vi "Launch p2.vi"(9 "Alias":string, 10 "Actor":refnum<class "Actor.lvclass">, 11 "jettl in":refnum<class "jettl.lvclass">) -> (0 "error out":errorcluster)   [LabVIEW 2021, in "jettl.lvlib" / "jettl.lvclass"]
uses:
  jettl.lvclass
  Actor/Actor/Actor.lvclass
  Create Wrapper.vi
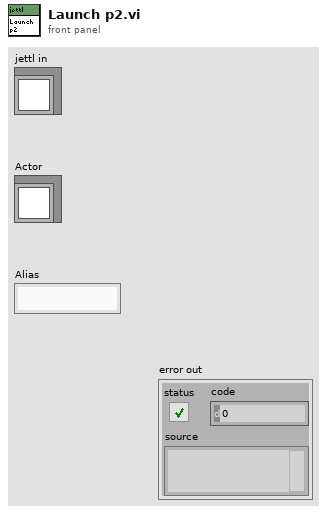
[diagram p1: front panel]
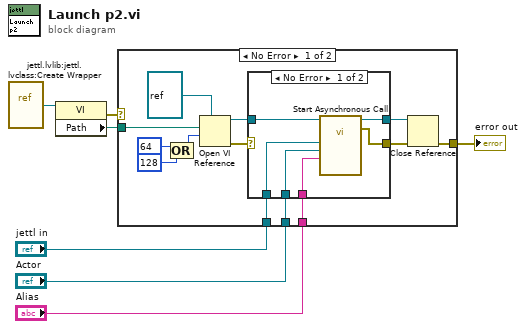
[diagram p0: block diagram]
diagram:
  n1 = vi-ref "jettl.lvlib:jettl.lvclass:Create Wrapper.vi"() -> (w6:refnum<vi>)
  n2 = property class="VI"(reference=w6) -> (error out=w7:errorcluster, "Path"=w5:path)  [unwired: 1 in, 1 out]
  n3 = case shown="No Error" w7 {
    selector: w7 -> [_ w29]
    tunnel: [w18 w29] -> w2
    tunnel: w5 -> [w14 _]
    tunnel: "Alias" -> [w10 _]
    tunnel: "Actor" -> [w9 _]
    tunnel: "jettl in" -> [w8 _]
    frame No Error {
      n4 = Compound Arithmetic op=OR(64 ("options: Multiple Clones,\n  Fire & Forget"), 128 ("options: Multiple Clones,\n  Fire & Forget")) -> (w16:i32)
      n5 = Open VI Reference(type specifier VI Refnum (for type only)=refnum<vi> refnum, vi path=w14, options=w16) -> (vi reference=w12:refnum<vi>, error out=w13:errorcluster)  [unwired: 3 in]
      n6 = case shown="No Error" w13 {
        selector: w13 -> [_ w28]
        tunnel: [w26 w27] -> w20
        tunnel: [w25 w28] -> w19
        tunnel: w12 -> [w24 w27]
        tunnel: w10 -> [w23 _]
        tunnel: w9 -> [w22 _]
        tunnel: w8 -> [w21 _]
        frame No Error {
          n7 = call-by-ref "Start Asynchronous Call"(reference=w24, "Alias"=w23, "Actor"=w22, "jettl in"=w21) -> (reference out=w26:refnum<vi>, error out=w25:errorcluster)  [unwired: 9 in, 1 out]
        }
        frame Error {
        }
      }
      n8 = Close Reference(reference=w20, error in (no error)=w19) -> (error out=w18:errorcluster)
    }
    frame Error {
    }
  }
  "error out" <- w2
